vi "Write Header Contents Class.vi"(8 "error in (no error)":errorcluster, 10 "Header Contents.lvclass":refnum<class "Header Contents.lvclass">, 11 "Simulated_Header in":refnum<class "Simulated_Header.lvclass">) -> (0 "error out":errorcluster, 3 "Simulated_Header out":refnum<class "Simulated_Header.lvclass">)   [LabVIEW 2018, in "Simulated_Header.lvclass"]
uses:
  Simulated_Header.lvclass
  Header Contents/Header Contents.lvclass
  Simulated_Header.lvclass/Simulated_Header.ctl
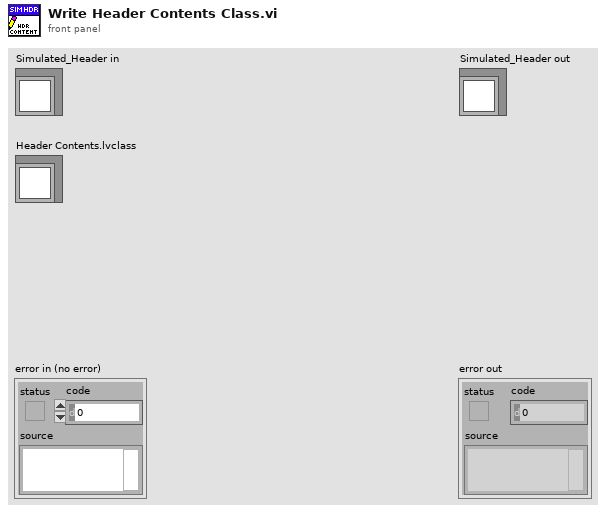
[diagram p1: front panel]
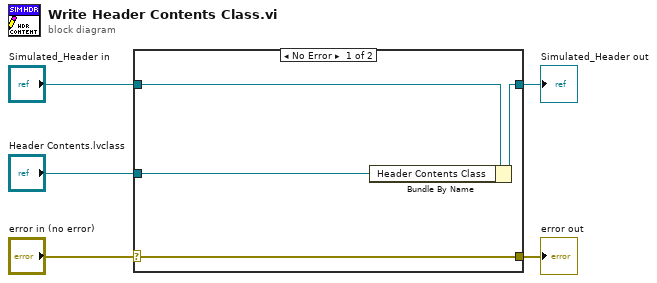
[diagram p0: block diagram]
diagram:
  n1 = case shown="No Error" "error in (no error)" {
    selector: "error in (no error)" -> [w9 w10]
    tunnel: [w9 w10] -> w4
    tunnel: [w7 w11] -> w2
    tunnel: "Simulated_Header in" -> [w8 w11]
    tunnel: "Header Contents.lvclass" -> [w6 _]
    frame No Error {
      n2 = Bundle By Name(cluster=w8, "Header Contents Class"=w6) -> (w7:refnum<class "Simulated_Header.lvclass">)
    }
    frame Error {
    }
  }
  "error out" <- w4
  "Simulated_Header out" <- w2
